vi "main.vi"() -> ()   [LabVIEW 2022 SP3]
uses:
  790827a8-57f0-3fcc-c817-03a3ff7fd63f.vi
panel:
  in  "Numeri totali":i32=100
  out "array w/ subset deleted":dbl[](array[numeric])
  out "Array di numeri primi":dbl[](array[numeric])
  out "Array iniziale":dbl[](array[numeric])
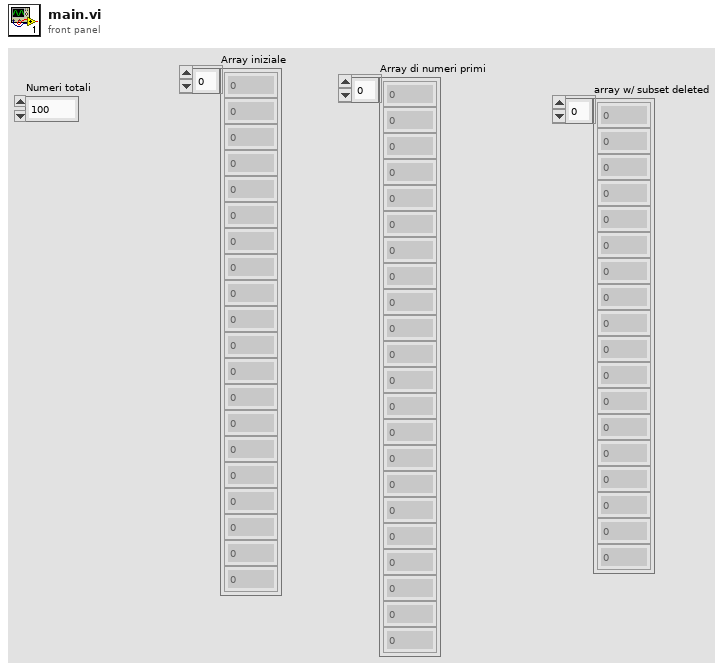
[diagram p1: front panel]
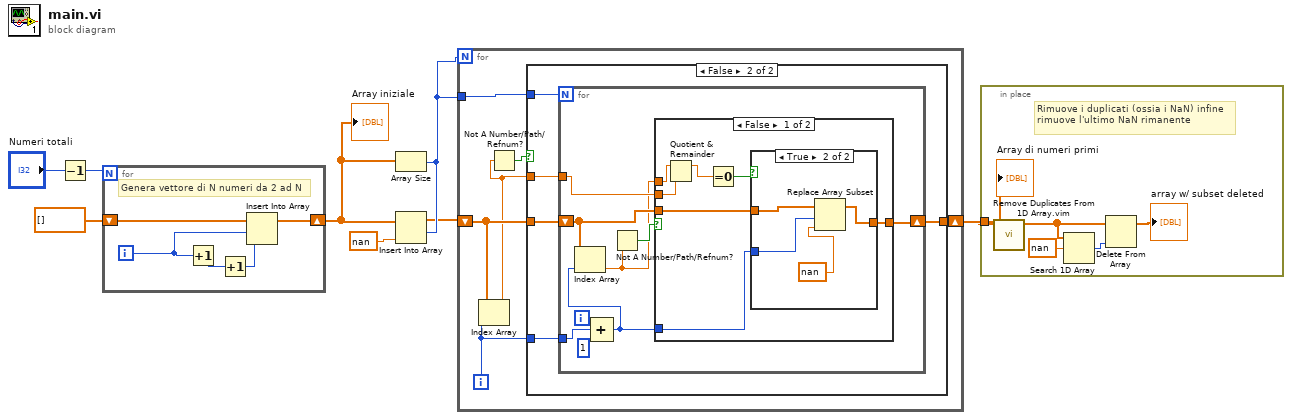
[diagram p0: block diagram]
diagram:
  n1 = Decrement(x="Numeri totali") -> (x-1=w7:i32)
  n2 = for {
    N: w7 -> [_]
    shift-right: [w12] -> w5
    shift-left: dbl[] [] ("array") -> [w13]
    i -> [w11]
    # "Genera vettore di N numeri da 2 ad N"
    n3 = Increment(x=w11) -> (x+1=w9:i32)
    n4 = Increment(x=w9) -> (x+1=w10:i32)
    n5 = Insert Into Array(array=w13, index=w11, new element=w10) -> (w12:dbl[])
  }
  "Array iniziale" <- w5
  n6 = Array Size(array=w5) -> (size(s)=w3:i32)
  n7 = Insert Into Array(array=w5, index=w3, new element=nan) -> (w2:dbl[])
  n8 = for {
    N: w3 -> [_]
    shift-right: [w19] -> w1
    shift-left: w2 -> [w18]
    tunnel: w3 -> [w16]
    i -> [w17]
    n9 = Index Array(array=w18, index=w17) -> (element=w15:dbl)
    n10 = Not A Number/Path/Refnum?(number/path/refnum=w15) -> (NaN/Path/Refnum?=w14:bool)
    n11 = case shown="False" w14 {
      tunnel: [w20 w25] -> w19
      tunnel: w18 -> [w20 w24]
      tunnel: w17 -> [_ w23]
      tunnel: w16 -> [_ w22]
      tunnel: w15 -> [_ w21]
      frame True {
      }
      frame False {
        n12 = for {
          N: w22 -> [_]
          shift-right: [w33] -> w25
          shift-left: w24 -> [w34]
          tunnel: w21 -> [w32]
          tunnel: w23 -> [w31]
          i -> [w30]
          n13 = Compound Arithmetic op=ADD(w30, w31, 1 ("value")) -> (w29:i32)
          n14 = Index Array(array=w34, index=w29) -> (element=w26:dbl)
          n15 = Not A Number/Path/Refnum?(number/path/refnum=w26) -> (NaN/Path/Refnum?=w27:bool)
          n16 = case shown="False" w27 {
            tunnel: w26 -> [w41 _]
            tunnel: w34 -> [w39 w47]
            tunnel: [w38 w47] -> w33
            tunnel: w32 -> [w36 _]
            tunnel: w29 -> [w35 _]
            frame False {
              n17 = Quotient & Remainder(x=w41, y=w36) -> (x-y*floor(x/y)=w37:dbl)  [unwired: 1 out]
              n18 = Equal To 0?(x=w37) -> (x = 0?=w40:bool)
              n19 = case shown="True" w40 {
                tunnel: w39 -> [w42 w45]
                tunnel: [w42 w46] -> w38
                tunnel: w35 -> [_ w44]
                frame False {
                }
                frame True {
                  n20 = Replace Array Subset(array=w45, new element=nan, index=w44) -> (w46:dbl[])
                }
              }
            }
            frame True {
            }
          }
        }
      }
    }
  }
  n21 = in-place {
    in-place-border: w1 -> [w52]
    # "Rimuove i duplicati (ossia i NaN) infine \nrimuove l'ultimo NaN rimanente"
    n22 = call "Remove Duplicates From 1D Array.vim"("array"=w52) -> ("array with duplicates removed"=w50:dbl[])  [unwired: 10 in]
    n23 = Search 1D Array(1D array=w50, element=nan) -> (index of element=w49:i32)  [unwired: 1 in]
    n24 = Delete From Array(array=w50, index=w49) -> (array with subset deleted=→"array w/ subset deleted":dbl[])  [unwired: 1 in, 1 out]
    "Array di numeri primi" <- w52
  }
